vi "HISTORY_RECORDER_EPICS.vi"() -> ()   [LabVIEW 2019]
uses:
  <vilib>/Platform/TimedLoop/XDataNode/timing_clust.ctl
  <vilib>/Platform/TimedLoop/XDataNode/nitl_modes.ctl
  <vilib>/Platform/TimedLoop/XDataNode/wakeup.ctl
  <vilib>/Utility/config.llb/Read Key (String).vi
  <userlib>/caLab/Private/Get_PV-1D.vi
  <vilib>/platform/TimedLoop/XDataNode/XDataNode.xnode
  <vilib>/Utility/config.llb/NI_LVConfig.lvlib
  <vilib>/Platform/TimedLoop/XDataNode/XDNodeRunTimeDep.lvlib
panel:
  out "Error":errorcluster
  out "HISTORY:maindir":string="P:\\BL13-0\\BL13-2\\HISTORY\\"
  out "BL132:CONFIG":path=path "S:/INI/BL132.INI"
  out "HISTORY file":path=path "P:/b_ogasawara/BL13-0/BL13-2/HISTORY/171103.csv"
  out "current time":timestamp
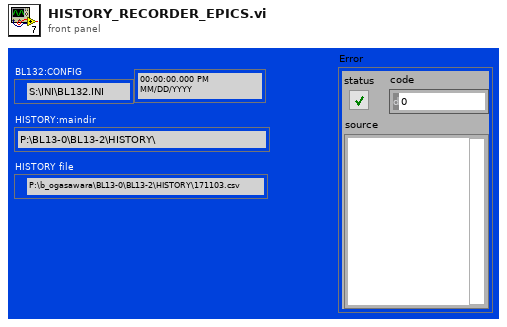
[diagram p1: front panel]
types:
  T1 = typedef "NI_LVConfig.lvlib/Config Data RefNum.ctl" = refnum<k1>
  T2 = typedef "XDNodeRunTimeDep.lvlib/timing_clust.ctl" = cluster{"Expected End [f-1]":u64, "Actual End [f-1]":u64, "Finished Late? [f-1]":bool, "Expected End [i-1]":u64, "Actual End [i-1]":u64, "Finished Late? [i-1]":bool, "Expected Start [i]":u64, "Actual Start [i]":u64, "Expected Start [f]":u64, "Actual Start [f]":u64, "Source Name":string, "Structure Name":string, "Period":i64, "Deadline":i64, "Offset":i64, "Start":i64, "Priority":i32, "Timeout":i32, "Mode":T3, "Wakeup Reason":T4, "Error":errorcluster, "Source Type":string, "Secondary Source Type":string, "Global End Time":u64, "Global Start Time":u64, "Frame Duration":u64, "Iteration Duration":u64, "Assigned CPU":i32, "I/O Scan Engine Mode":u32}
  T3 = typedef "XDNodeRunTimeDep.lvlib/nitl_modes.ctl" = enum32{"No Change", "Process missed periods, maintain original phase", "Discard missed periods, maintain original phase", "Process missed periods, ignore original phase", "Discard missed periods, ignore original phase"}
  T4 = typedef "XDNodeRunTimeDep.lvlib/wakeup.ctl" = enum32{"Normal", "Aborted", "Asynchronous wakeup", "Timing source error", "Timed loop error", "Timeout"}
  T5 = enum16{"open", "replace", "create", "open or create", "replace or create", "replace or create with confirmation"}
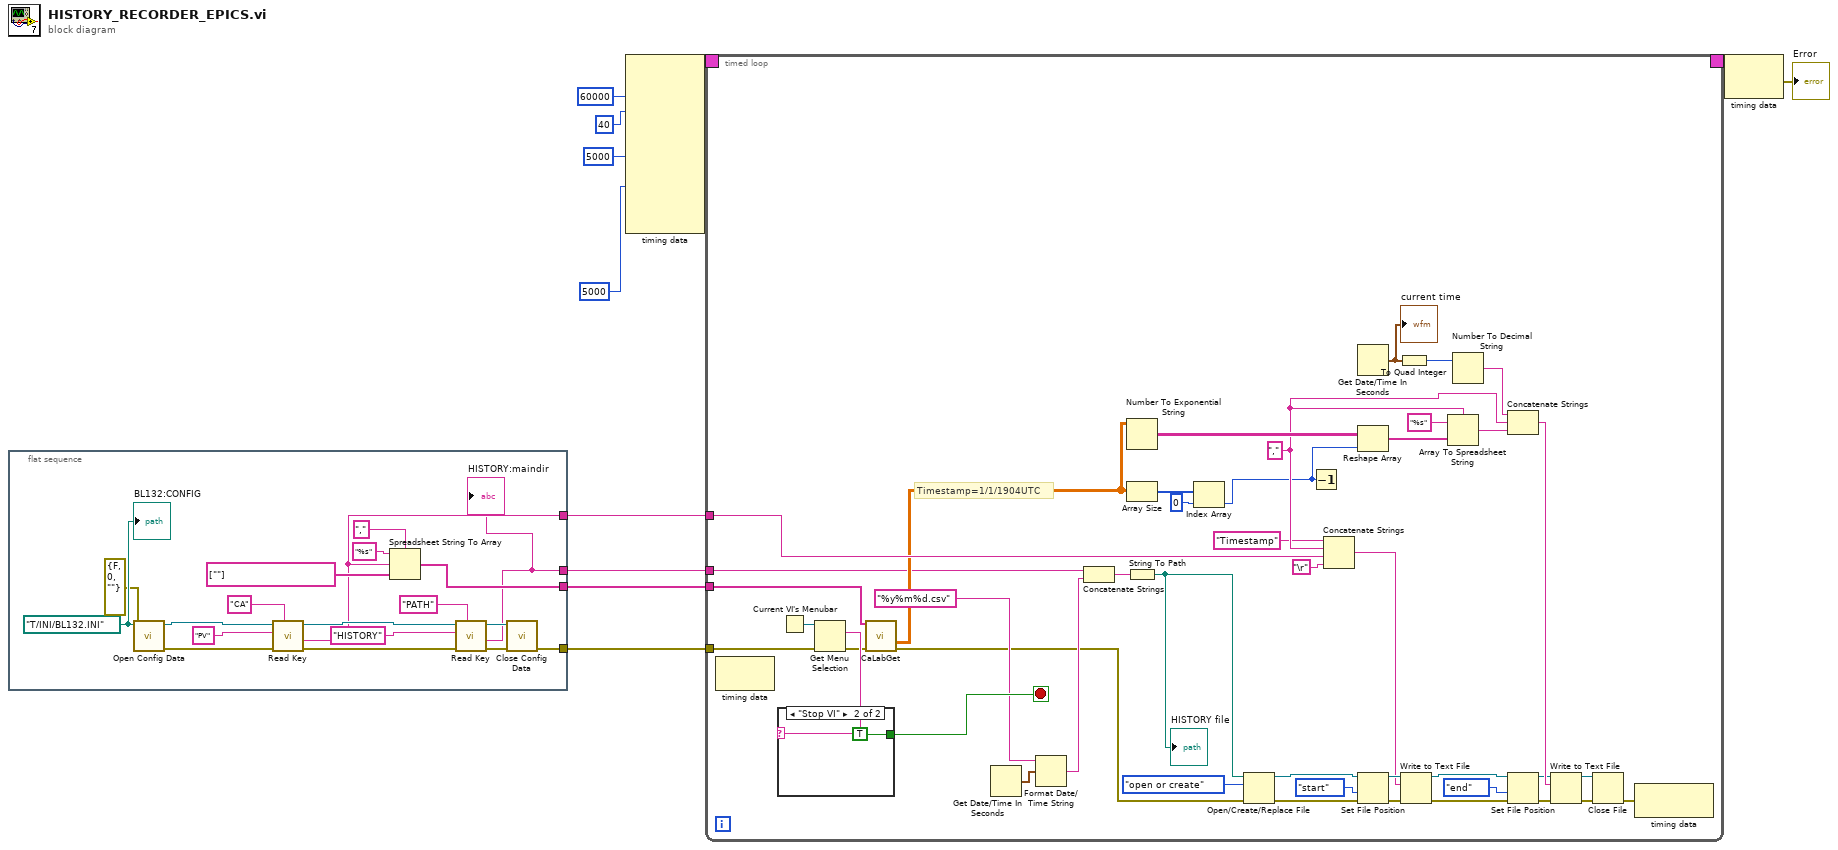
[diagram p0: block diagram]
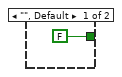
[diagram p2: hidden frame]
diagram:
  n1 = flat-sequence {
    tunnel: [w20] -> w8
    tunnel: [w18] -> w7
    tunnel: [w14] -> w3
    tunnel: [w12] -> w2
    frame #0 {
      w29 = path "T:/INI/BL132.INI" ("configuration file path")
      n2 = call <vilib>:"Open Config Data.vi"("error in (no error)"=errorcluster {"status"=FALSE, "code"=0, "source"=""}, "configuration file path"=w29) -> ("error out"=w15:errorcluster, "refnum"=w26:T1)  [unwired: 7 in, 1 out]
      n3 = call-poly <vilib>:"Read Key.vi"("section"="CA", "error in (no error)"=w15, "key"="PV", "refnum"=w26) -> ("error out"=w16:errorcluster, "value"=w18:string, "refnum out"=w21:T1)  [unwired: 4 in, 1 out]
      n4 = Spreadsheet String To Array(delimiter (Tab)=",", format string="%s", spreadsheet string=w18, array type (2D Dbl)=string[] [""] ("Strings []")) -> (array=w20:string[])
      n5 = call-poly <vilib>:"Read Key.vi"("section"="PATH" ("key"), "error in (no error)"=w16, "key"="HISTORY" ("section"), "refnum"=w21) -> ("error out"=w17:errorcluster, "value"=w12:string, "refnum out"=w30:T1)  [unwired: 4 in, 1 out]
      "HISTORY:maindir" <- w12
      n6 = call <vilib>:"Close Config Data.vi"("error in (no error)"=w17, "refnum"=w30) -> ("error out"=w14:errorcluster)  [unwired: 8 in, 1 out]
      "BL132:CONFIG" <- w29
    }
  }
  n7 = node-c288(i64 60000 ("Period"), 40 ("Priority"), i64 5000 ("Deadline"), 5000 ("Timeout")) -> (w11:T2)  [unwired: 6 in]
  n8 = timed-loop {
    timing: w11 -> [_]
    timing-out: [_] -> w10
    tunnel: w8 -> [w62]
    tunnel: w7 -> [w47]
    tunnel: w3 -> [w35]
    tunnel: w2 -> [w31]
    stop <- w72 stop-if-true
    w49 = "," ("string")
    # "Timestamp=1/1/1904UTC"
    n9 = node-c288() -> ()  [unwired: 1 in, 1 out]
    n10 = Current VI's Menubar() -> (w74:refnum<k9>)
    n11 = Get Menu Selection(0:w74, 3:w35) -> (6:w73:string, 8:w34:errorcluster)  [unwired: 2 in, 3 out]
    n12 = case shown="\"Stop VI\"" w73 {
      tunnel: [FALSE TRUE] -> w72
      frame "", Default {
      }
      frame "Stop VI" {
      }
    }
    n13 = call-poly <userlib>:"CaLabGet.vi"("PV Names"=w62, "Error in (no error)"=w34) -> ("Value Array (number)"=w44:dbl[][], "Error out"=w33:errorcluster)  [unwired: 7 in, 5 out]
    n14 = Get Date/Time In Seconds() -> (seconds since 1Jan1904=w54:timestamp)
    n15 = Format Date/Time String(time format string (%c)="%y%m%d.csv", seconds (now)=w54) -> (date/time string=w56:string)  [unwired: 1 in]
    n16 = Concatenate Strings(w31, w56) -> (w57:string)
    n17 = Number To Exponential String(number=w44) -> (E-format string=w70:string[][])  [unwired: 3 in]
    n18 = Array Size(array=w44) -> (size(s)=w43:i32[])
    n19 = String To Path(string=w57) -> (path=w58:path)
    "HISTORY file" <- w58
    n20 = Index Array(array=w43, index=0 ("dimension size")) -> (element=w32:i32)
    n21 = Open/Create/Replace File(file path (use dialog)=w58, error in=w33, operation (0:open)=T5."open or create" ("operation (0:open) 2")) -> (refnum out=w52:refnum<file>, error out=w36:errorcluster)  [unwired: 3 in, 1 out]
    n22 = Decrement(x=w32) -> ()  [unwired: 1 out]
    n23 = Concatenate Strings("Timestamp" ("format string"), w49, w47, "\r") -> (w46:string)
    n24 = Get Date/Time In Seconds() -> (seconds since 1Jan1904=w71:timestamp)
    "current time" <- w71
    n25 = Reshape Array(w70, w32) -> (w69:string[])
    n26 = Set File Position(refnum=w52, from (0:start)=enum16{"start", "end", "current"}."start", error in=w36) -> (refnum out=w51:refnum<file>, error out=w38:errorcluster)  [unwired: 1 in]
    n27 = To Quad Integer(1:w71) -> (0:w66:i64)
    n28 = Write to Text File(file (use dialog)=w51, text=w46, error in=w38) -> (refnum out=w50:refnum<file>, error out=w37:errorcluster)  [unwired: 1 in, 1 out]
    n29 = Array To Spreadsheet String(delimiter (Tab)=w49, array=w69, 3:"%s" ("format string")) -> (spreadsheet string=w67:string)
    n30 = Number To Decimal String(number=w66) -> (decimal integer string=w65:string)  [unwired: 1 in]
    n31 = Concatenate Strings(w65, w49, w67) -> (w64:string)
    n32 = Set File Position(refnum=w50, from (0:start)=enum16{"start", "end", "current"}."end", error in=w37) -> (refnum out=w60:refnum<file>, error out=w41:errorcluster)  [unwired: 1 in]
    n33 = Write to Text File(file (use dialog)=w60, text=w64, error in=w41) -> (refnum out=w63:refnum<file>, error out=w40:errorcluster)  [unwired: 1 in, 1 out]
    n34 = Close File(refnum=w63, error in=w40) -> (error out=w39:errorcluster)  [unwired: 1 out]
    n35 = node-c288(w39) -> ()  [unwired: 1 out]
  }
  n36 = node-c288(w10) -> (→"Error":errorcluster)
